vi "Close TCP Connection.vi"(8 "error in (no error)":errorcluster, 11 "TCP Network Connection in":refnum<k5>) -> (0 "error out":errorcluster)   [LabVIEW 2019, in "TimingDRV System Explorer.lvlib"]
uses:
  TimingDRV System Explorer.lvlib
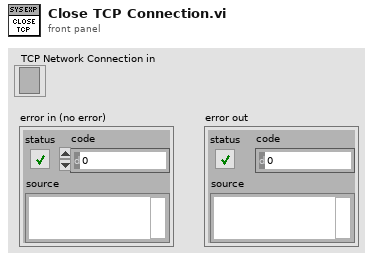
[diagram p1: front panel]
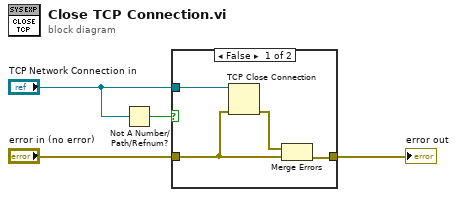
[diagram p0: block diagram]
diagram:
  n1 = Not A Number/Path/Refnum?(number/path/refnum="TCP Network Connection in") -> (NaN/Path/Refnum?=w1:bool)
  n2 = case shown="False" w1 {
    tunnel: "error in (no error)" -> [w7 w9]
    tunnel: [w5 w9] -> w3
    tunnel: "TCP Network Connection in" -> [w8 _]
    frame False {
      n3 = TCP Close Connection(connection ID=w8, error in (no error)=w7) -> (error out=w6:errorcluster)  [unwired: 1 in, 1 out]
      n4 = Merge Errors(w6, w7) -> (w5:errorcluster)
    }
    frame True {
    }
  }
  "error out" <- w3
